vi "FFT.vi"() -> ()   [LabVIEW 2018]
uses:
  <vilib>/measure/maspectr.llb/FFT Power Spectrum for N Chan.vi
  <vilib>/measure/NI_MAPro.lvlib
panel:
  in  "Data window":T1={"Start"=200000, "Length"=500000, "Channel numbers"=[0], "Cannel names"=["V"], "Group name"="p"}
  out "Signal graph":waveform(dbl)[](graph)
  in  "Preserve old data":bool
  out "FFT Graph":cluster{"f0":dbl, "df":dbl, "magnitude":dbl[]}[](graph)
  in  "Data File Type":T2(ring)
  in  "Window":u32(ring)=1 items=["Rectangle"=0, "Hanning"=1, "Hamming"=2, "Blackman-Harris"=3, "Exact Blackman"=4, "Blackman"=5, "Flat Top"=6, "4 Term B-Harris "=7, "7 Term B-Harris"=8, "Low Sidelobe"=9, "Blackman Nuttall"=11, "Triangle"=30, "Bartlett-Hanning"=31, "Bohman"=32, "Parzen"=33, "Welch"=34, "Kaiser"=60, "Dolph-Chebyshev"=61, "Gaussian"=62]
  in  "Input file path":path
  # "OR"
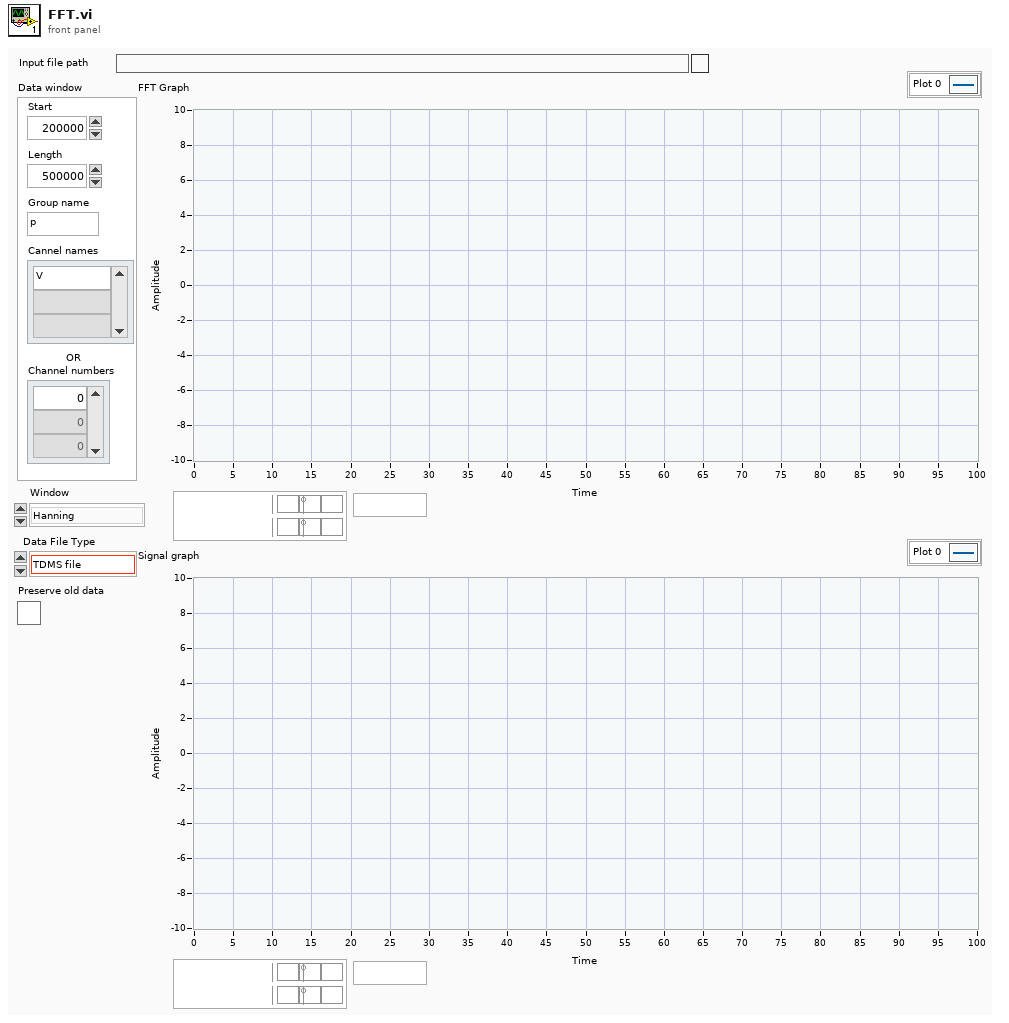
[diagram p1: front panel]
types:
  T1 = cluster{"Start":i64, "Length":i32, "Channel numbers":i64[], "Cannel names":string[], "Group name":string}
  T2 = enum16{"TDMS file", "Tektronics ISF", "BinF file", "ASCII File", "BinH File", "BinW File", "BINARY File"}
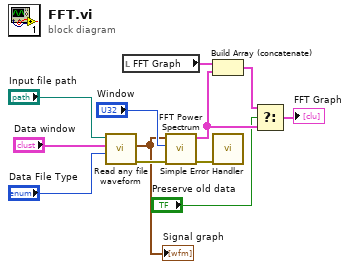
[diagram p0: block diagram]
diagram:
  n1 = call "Read any file waveform.vi"("Data File Type"="Data File Type", "Data window"="Data window", "Input file path"="Input file path") -> ("error out"=w11:errorcluster, "Data out"=w3:waveform(dbl)[])  [unwired: 4 in, 3 out]
  "Signal graph" <- w3
  n2 = local read "FFT Graph"() -> (w9:cluster{"f0":dbl, "df":dbl, "magnitude":dbl[]}[])
  n3 = call-poly <vilib>:"FFT Power Spectrum.vi"("error in (no error)"=w11, "window"="Window", "time signals"=w3) -> ("error out"=w1:errorcluster, "power spectra"=w7:cluster{"f0":dbl, "df":dbl, "magnitude":dbl[]}[])  [unwired: 3 in, 4 out]
  n4 = Build Array (concatenate)(w9, w7) -> (w8:cluster{"f0":dbl, "df":dbl, "magnitude":dbl[]}[])
  n5 = call <vilib>:"Simple Error Handler.vi"("error in (no error)"=w1) -> ()  [unwired: 4 in, 5 out]
  n6 = Select(t=w8, s="Preserve old data", f=w7) -> (s? t:f=→"FFT Graph":cluster{"f0":dbl, "df":dbl, "magnitude":dbl[]}[])
